vi "Close Application Style Reference.vi"(8 "error in (no error)":errorcluster, 11 "Application Style Reference":T1) -> (0 "error out":errorcluster)   [LabVIEW 2015, in "IViewable.lvlib" / "ApplicationStyleReference.lvclass"]
uses:
  ApplicationStyleReference.lvclass
  Application Style Reference.ctl
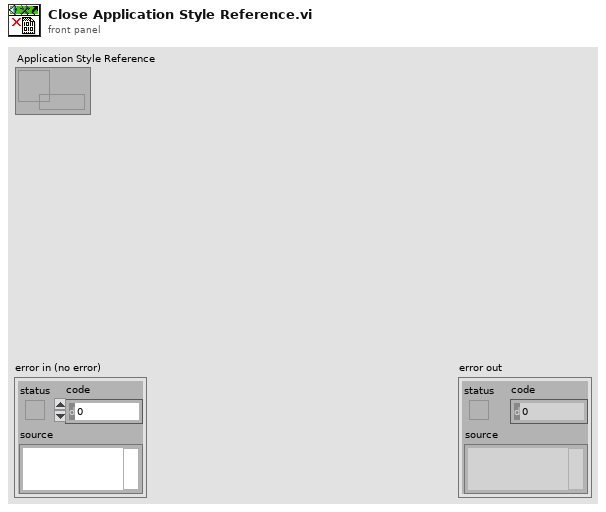
[diagram p1: front panel]
types:
  T1 = typedef "IViewable.lvlib/ApplicationStyleReference.lvclass/Application Style Reference.ctl" = refnum<data-value>
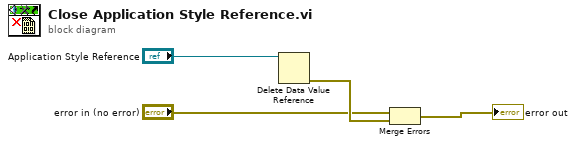
[diagram p0: block diagram]
diagram:
  n1 = Delete Data Value Reference(data value reference="Application Style Reference") -> (error out=w3:errorcluster)  [unwired: 1 in, 1 out]
  n2 = Merge Errors("error in (no error)", w3) -> (→"error out":errorcluster)
